vi "Handle Errors.vi"(8 "error in (no error)":errorcluster, 10 "Location":string, 11 "Error Handler Interface In":refnum<class "Mock Error Handler Interface.lvclass">) -> (0 "error out":errorcluster, 3 "Error Handler Interface Out":refnum<class "Mock Error Handler Interface.lvclass">)   [LabVIEW 2020, in "Mock Error Handler Interface.lvclass"]
doc: "The implementation of this VI defines how errors are handled."
uses:
  Mock Error Handler Interface.lvclass
  C:/Program Files (x86)/National Instruments/LabVIEW 2020/vi.lib/Astemes/LMock/Mock.lvclass
  <vilib>/Astemes/LMock/Mock.lvclass
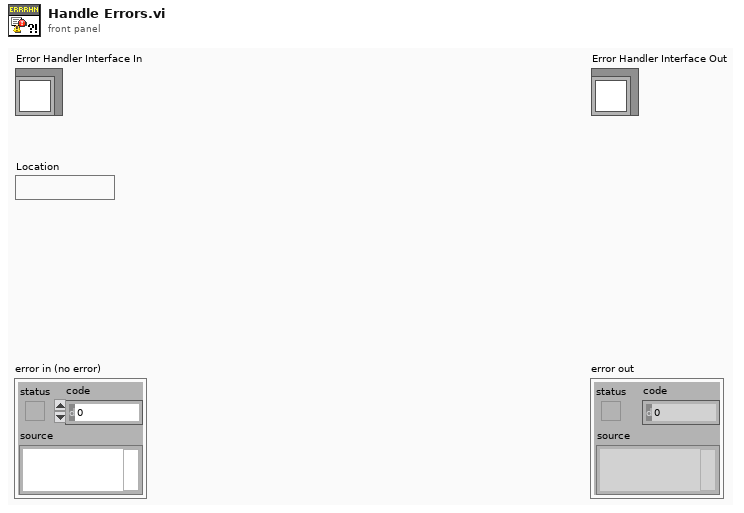
[diagram p1: front panel]
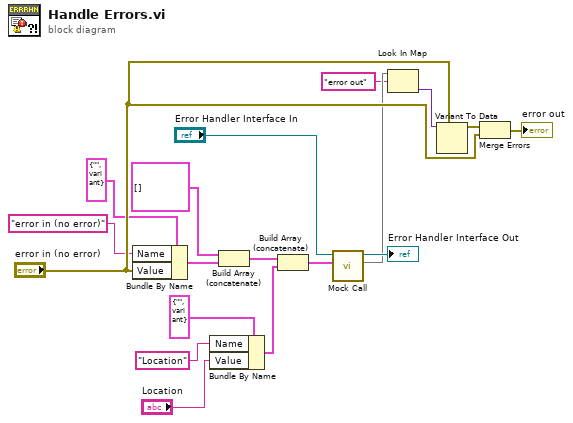
[diagram p0: block diagram]
diagram:
  n1 = Bundle By Name(cluster=cluster{"Name":string, "Value":variant} {"Name"="", "Value"=variant} ("element"), "Name"="error in (no error)", "Value"="error in (no error)") -> (w3:cluster{"Name":string, "Value":variant})
  n2 = Bundle By Name(cluster=cluster{"Name":string, "Value":variant} {"Name"="", "Value"=variant} ("element"), "Name"="Location", "Value"="Location") -> (w1:cluster{"Name":string, "Value":variant})
  n3 = Build Array (concatenate)(cluster{"Name":string, "Value":variant}[] [] ("Control Values"), w3) -> (w12:cluster{"Name":string, "Value":variant}[])
  n4 = Build Array (concatenate)(w12, w1) -> (w15:cluster{"Name":string, "Value":variant}[])
  n5 = call <vilib>:"Mock Call.vi"("Control Values"=w15, "Mock In"="Error Handler Interface In") -> ("Return Values"=w10:map{string, variant}, "Mock Out"=→"Error Handler Interface Out":refnum<class "Mock Error Handler Interface.lvclass">)  [unwired: 8 in]
  n6 = Look In Map(map=w10, key="error out") -> (value=w8:variant)  [unwired: 1 in, 1 out]
  n7 = Variant To Data(type="error in (no error)", Variant=w8) -> (data=w7:errorcluster)  [unwired: 1 in, 1 out]
  n8 = Merge Errors(w7, "error in (no error)") -> (→"error out":errorcluster)
